vi "OAT Remove Slow Roll Error.vi"   [LabVIEW 2017]
doc: "Performs run out compensation for proximity probe signals. This vi receives <B>magnitudes (RMS)</B> and <B>phase lags</B> from the order tracking vis and the <B>slow roll vectors</B> of the same orders.It removes the slow roll errors by subtracting the <B>slow roll vectors</B> from the corresponding <B>magnitudes (RMS)</B> and <B>phase lags</B>."
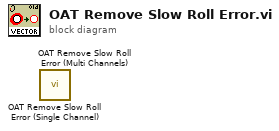
[diagram p0: block diagram]
diagram:
  n1 = call <vilib>:"OAT Remove Slow Roll Error (Single Channel).vi"() -> ()  [unwired: 8 in, 4 out]
  n2 = call <vilib>:"OAT Remove Slow Roll Error (Multi Channels).vi"() -> ()  [unwired: 8 in, 4 out]
